vi "Query Ethernet Setup.vi"(8 "error in (no error)":errorcluster, 11 "VISA resource name":refnum<visa-resource-name>) -> (0 "error out":errorcluster, 1 "IP Address":string, 2 "IP Setup Mode":u16(ring) items=["Auto", "Manual"], 3 "VISA resource name out":refnum<visa-resource-name>, 4 "Subnet Mask":string, 5 "Device Name":string, 6 "Gateway IP":string)   [LabVIEW 2016, in "APT 300XAC Series.lvlib"]
doc: "Queries the IP Settings for the power source instrument.\n1. Device Name\n2. IP Setup Mode\n3. IP Address\n4. Subnet Mask\n5. Gateway IP"
uses:
  APT 300XAC Series.lvlib
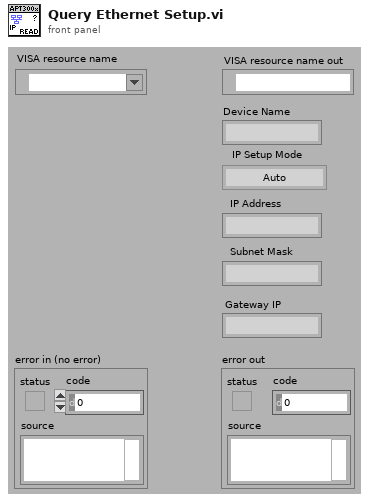
[diagram p1: front panel]
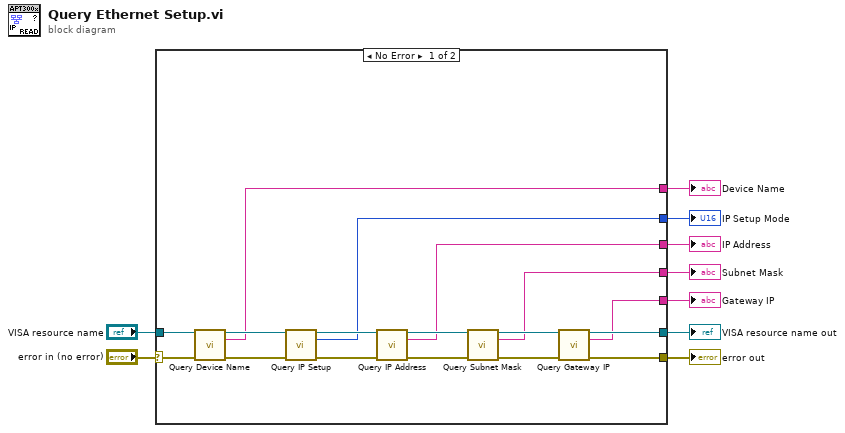
[diagram p0: block diagram]
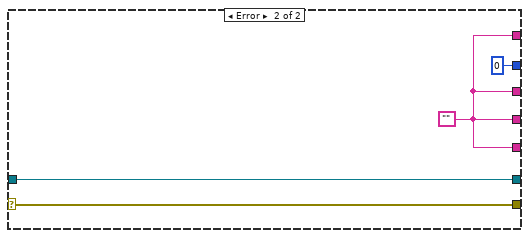
[diagram p2: hidden frame]
diagram:
  n1 = case shown="No Error" "error in (no error)" {
    selector: "error in (no error)" -> [w25 w30]
    tunnel: "VISA resource name" -> [w26 w29]
    tunnel: [w18 w30] -> w8
    tunnel: [w19 w29] -> w7
    tunnel: [w14 w27] -> w5
    tunnel: [w13 u16 0 ("Mode")] -> w4
    tunnel: [w12 w27] -> w3
    tunnel: [w11 w27] -> w2
    tunnel: [w10 w27] -> w1
    frame No Error {
      n2 = call "Query Device Name.vi"("VISA resource name"=w26, "error in (no error)"=w25) -> ("VISA resource name out"=w24:refnum<visa-resource-name>, "Device Name"=w14:string, "error out"=w23:errorcluster)  [unwired: 11 in]
      n3 = call "Query IP Setup.vi"("VISA resource name"=w24, "error in (no error)"=w23) -> ("VISA resource name out"=w22:refnum<visa-resource-name>, "IP Setup Mode"=w13:u16, "error out"=w15:errorcluster)  [unwired: 11 in]
      n4 = call "Query IP Address.vi"("VISA resource name"=w22, "error in (no error)"=w15) -> ("VISA resource name out"=w21:refnum<visa-resource-name>, "IP Address"=w12:string, "error out"=w16:errorcluster)  [unwired: 11 in]
      n5 = call "Query Subnet Mask.vi"("VISA resource name"=w21, "error in (no error)"=w16) -> ("VISA resource name out"=w20:refnum<visa-resource-name>, "Subnet Mask"=w11:string, "error out"=w17:errorcluster)  [unwired: 11 in]
      n6 = call "Query Gateway IP.vi"("VISA resource name"=w20, "error in (no error)"=w17) -> ("VISA resource name out"=w19:refnum<visa-resource-name>, "Gateway IP"=w10:string, "error out"=w18:errorcluster)  [unwired: 11 in]
    }
    frame Error {
      w27 = ""
    }
  }
  "VISA resource name out" <- w7
  "error out" <- w8
  "Device Name" <- w5
  "IP Setup Mode" <- w4
  "IP Address" <- w3
  "Subnet Mask" <- w2
  "Gateway IP" <- w1
